vi "get_time_string.vi"() -> (0 "date/time string":string)   [LabVIEW 2019, in "Log.lvlib" / "Log.lvclass"]
uses:
  Log.lvclass
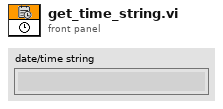
[diagram p1: front panel]
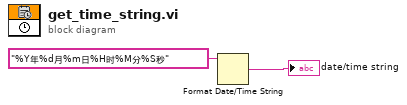
[diagram p0: block diagram]
diagram:
  n1 = Format Date/Time String(time format string (%c)="%Y年%d月%m日%H时%M分%S秒" ("时间格式字符串(%c)")) -> (date/time string=→"date/time string":string)  [unwired: 2 in]
